vi "UART 8N1 Read FIFO.vi"(8 "Error In":errorcluster, 9 "Timeout (ms)":i32=5000, 10 "Number of Elements":u32, 11 "FPGA VI Reference In":refnum<k20>) -> (0 "Error Out":errorcluster, 2 "Elements Remaining":u32)   [LabVIEW 2018]
uses:
  <vilib>/Utility/error.llb/Error Cluster From Error Code.vi
  <vilib>/rvi/errors/niLvFpgaAdjustHostInterfaceError.vi
  <vilib>/rvi/interface/nirviMethod/nirviMethod.xnode
  Program Files (x86)/National Instruments/LabVIEW 2018/instr.lib/niVST/FPGA/Templates/FPGA Bitfiles/niVSTFPGA_UART.lvbitx
  <vilib>/rvi/errors/niLvFpgaMergeErrorWithErrorCode.vi
  <vilib>/FPGAPlugInAG/PXIe-5840/niLvFpga_ReadFifo_PXIe-5840.vi
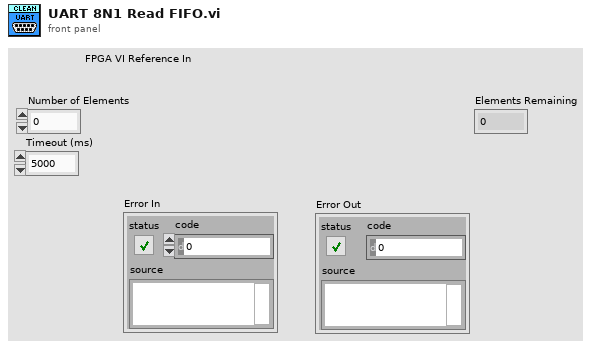
[diagram p1: front panel]
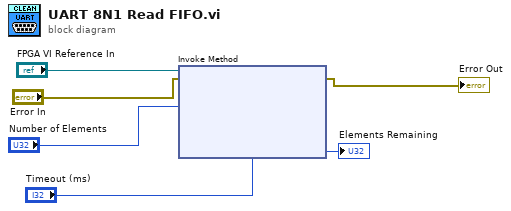
[diagram p0: block diagram]
diagram:
  n1 = xnode "Invoke Method"("FPGA VI Reference In"="FPGA VI Reference In", "error in"="Error In", "Number of Elements"="Number of Elements", "Timeout (ms)"="Timeout (ms)") -> ("error out"=→"Error Out":errorcluster, "Elements Remaining"=→"Elements Remaining":u32)  [unwired: 2 out]
